vi "Measure Current.vi"(8 "error in (no error)":errorcluster, 9 "Sample Rate":dbl=1000000.0, 11 "number of samples":i32=100) -> (0 "error out":errorcluster, 1 "read current (A)":dbl, 2 "read voltage (V)":dbl)   [LabVIEW 2019]
uses:
  <vilib>/DAQmx/read.llb/DAQmx Read (Analog 1D DBL 1Chan NSamp).vi
  Globals.vi
  <vilib>/DAQmx/create/channels.llb/DAQmx Create Channel (AI-Voltage-Basic).vi
  <vilib>/DAQmx/configure/timing.llb/DAQmx Timing (Sample Clock).vi
  <vilib>/DAQmx/miscellaneous.llb/DAQmx Fill In Error Info.vi
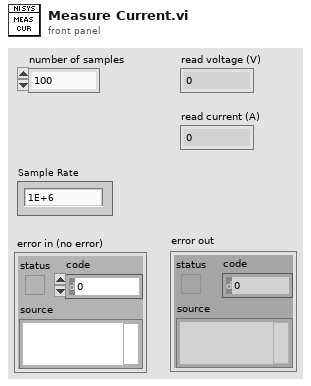
[diagram p1: front panel]
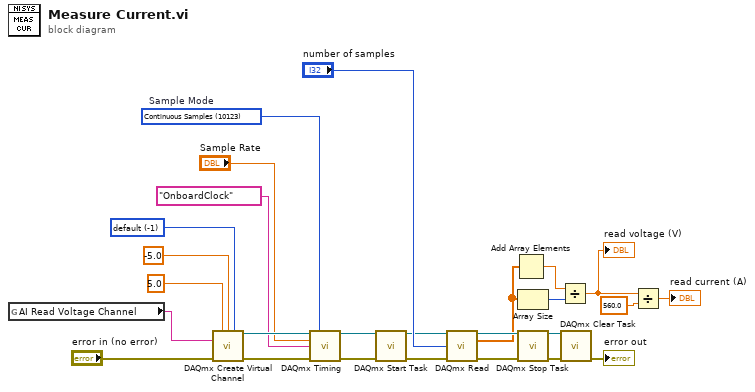
[diagram p0: block diagram]
diagram:
  w3 = -1 items=["default"=-1, "RSE"=10083, "NRSE"=10078, "Differential"=10106, "Pseudodifferential"=12529] ("Terminal Configuration 2")
  w6 = 10123 items=["Finite Samples"=10178, "Continuous Samples"=10123, "Hardware Timed Single Point"=12522]  # Sample Mode
  n1 = global read "Globals.vi" "AI Read Voltage Channel"() -> (w2:tag)
  n2 = call-poly <vilib>:"DAQmx Create Virtual Channel.vi"("maximum value"=5.0 ("Max Voltage 2"), "minimum value"=-5.0 ("Min Voltage 2"), "input terminal configuration"=w3, "physical channels"=w2, "error in"="error in (no error)") -> ("task out"=w10:refnum<k21>, "error out"=w9:errorcluster)  [unwired: 9 in]
  n3 = call-poly <vilib>:"DAQmx Timing.vi"("task/channels in"=w10, "sample mode"=w6, "rate"="Sample Rate", "source"=tag "OnboardClock" ("Sample Clock Source"), "error in"=w9) -> ("task out"=w11:refnum<k21>, "error out"=w12:errorcluster)  [unwired: 9 in]
  n4 = call <vilib>:"DAQmx Start Task.vi"("task/channels in"=w11, "error in"=w12) -> ("task out"=w13:refnum<k21>, "error out"=w14:errorcluster)  [unwired: 12 in]
  n5 = call-poly <vilib>:"DAQmx Read.vi"("task/channels in"=w13, "number of samples per channel"="number of samples", "error in"=w14) -> ("task out"=w24:refnum<k21>, "data"=w15:dbl[], "error out"=w26:errorcluster)  [unwired: 10 in]
  n6 = Add Array Elements(numeric array=w15) -> (sum=w17:dbl)
  n7 = Array Size(array=w15) -> (size(s)=w16:i32)
  n8 = call <vilib>:"DAQmx Stop Task.vi"("task/channels in"=w24, "error in"=w26) -> ("task out"=w23:refnum<k21>, "error out"=w25:errorcluster)  [unwired: 12 in]
  n9 = Divide(x=w17, y=w16) -> (x/y=w20:dbl)
  "read voltage (V)" <- w20
  n10 = call <vilib>:"DAQmx Clear Task.vi"("task in"=w23, "error in"=w25) -> ("error out"=→"error out":errorcluster)  [unwired: 13 in]
  n11 = Divide(x=w20, y=560.0) -> (x/y=→"read current (A)":dbl)
